vi "Send Send Packets.vi"(5 "Send Period (ms)":i32=1000, 7 "Priority":T1=enum."Normal" caption="Message Priority (Normal)", 8 "error in (no error)":errorcluster, 9 "Number of Packets":i32=1, 10 "Data To Send":string, 11 "Message Enqueuer in":refnum<class "Message Enqueuer.lvclass">) -> (0 "error out":errorcluster, 3 "Message Enqueuer out":refnum<class "Message Enqueuer.lvclass">)   [LabVIEW 2021, in "Echo Reply Test With Server Manager.lvlib" / "Send Packets Msg.lvclass"]
doc: "Sends the <b>Send Packets Msg.lvclass</b> message.\n\nThis message will call <b>Send Packets.vi</b> on the <b>Echo Broadcast Test With Server Manager.lvlib:WS Test Server Subscriber.lvclass</b> actor.\n\n<b>Send Packets.vi Description</b>"
uses:
  Send Packets Msg.lvclass
  Send Packets Msg.lvclass/Send Packets Msg.ctl
  <vilib>/ActorFramework/Message Enqueuer/Message Enqueuer.lvclass
  C:/Program Files/National Instruments/LabVIEW 2021/vi.lib/ActorFramework/Message/Message.lvclass
  C:/Projects/WebSocket-Actor/Examples/Echo Reply Test With Server Manager/WS Test Server Subscriber Messages/Send Packets Msg/Send Packets Msg.lvclass
  <vilib>/ActorFramework/Message Enqueuer/Message Priority.ctl
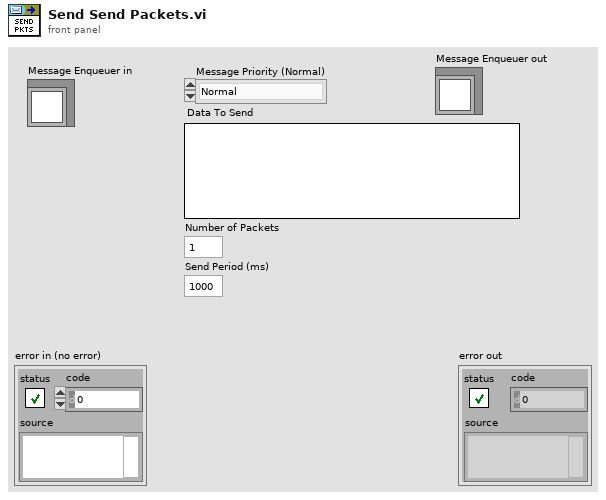
[diagram p1: front panel]
types:
  T1 = typedef "Actor Framework.lvlib/Message Enqueuer.lvclass/Message Priority.ctl" = enum16{"Low", "Normal", "High"}
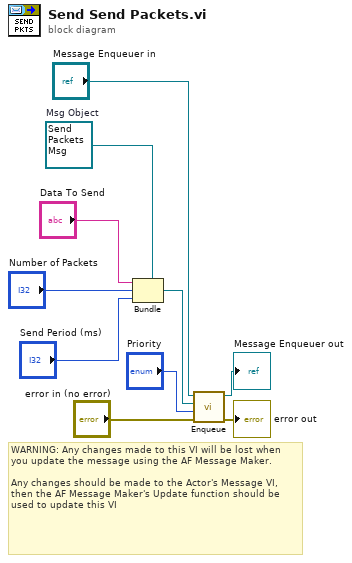
[diagram p0: block diagram]
diagram:
  w7 = refnum<class "Send Packets Msg.lvclass"> refnum  # Msg Object
  # "WARNING: Any changes made to this VI will be lost when you update the message using the AF Message Maker.\n\nAny changes should be made to the Actor's Message VI, then the AF Message Maker's Update function should be used to update this VI"
  n1 = Bundle(cluster=w7, "Data To Send", "Number of Packets", "Send Period (ms)") -> (w2:refnum<class "Send Packets Msg.lvclass">)
  n2 = call <vilib>:"Enqueue.vi"("error in (no error)"="error in (no error)", "Message Priority (Normal)"="Priority", "Message"=w2, "Message Enqueuer in"="Message Enqueuer in") -> ("error out"=→"error out":errorcluster, "Message Enqueuer in"=→"Message Enqueuer out":refnum<class "Message Enqueuer.lvclass">)  [unwired: 6 in]
